vi "Tcp Request.vi"(8 "error in (no error)":errorcluster, 9 "Timeout (0ms)":i32, 11 "Conn in":refnum<k5>) -> (0 "error out":errorcluster, 2 "WSGI Request":T1, 3 "Conn out":refnum<k5>)   [LabVIEW 2021, in "HttpServer.lvlib"]
uses:
  HttpServer.lvlib
  TypeDefs/WSGI.ctl
  <vilib>/Utility/error.llb/Error Cluster From Error Code.vi
  <vilib>/ErrorRing/Error Ring.xnode
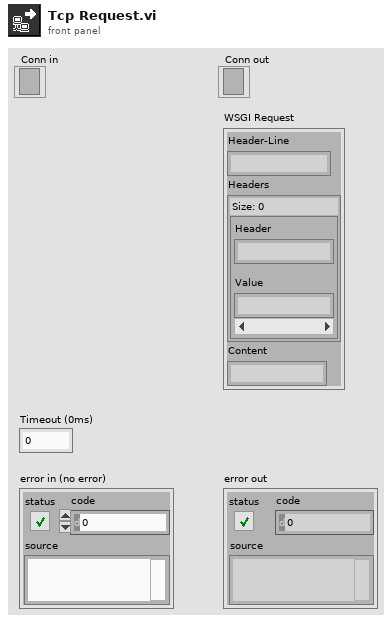
[diagram p1: front panel]
types:
  T1 = typedef "HttpServer.lvlib/WSGI.ctl" = cluster{"Header-Line":string, "Headers":map{string, string}, "Content":string}
  T2 = enum16{"Standard", "Buffered", "CRLF", "Immediate"}
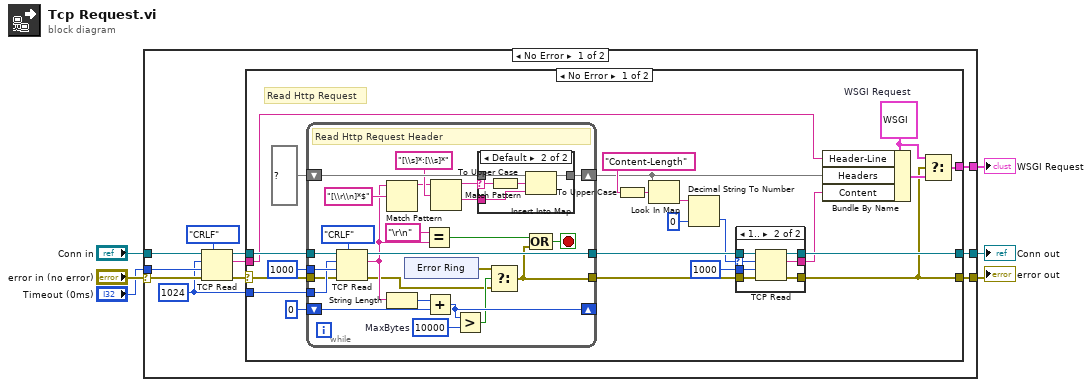
[diagram p0: block diagram]
diagram:
  n1 = case shown="No Error" "error in (no error)" {
    selector: "error in (no error)" -> [w15 w87]
    tunnel: [w17 w87] -> w6
    tunnel: [w16 w86] -> w5
    tunnel: "Conn in" -> [w12 w86]
    tunnel: "Timeout (0ms)" -> [w14 _]
    tunnel: [w13 _] -> w2
    frame No Error {
      w7 = 1024
      n2 = TCP Read(connection ID=w12, bytes to read=w7, error in (no error)=w15, 7:T2."CRLF" ("mode (standard)"), 9:w14) -> (connection ID out=w10:refnum<k5>, data out=w8:string, error out=w9:errorcluster)
      n3 = case shown="No Error" w9 {
        selector: w9 -> [w38 w85]
        tunnel: w10 -> [w39 w84]
        tunnel: w8 -> [w37 _]
        tunnel: w7 -> [w36 _]
        tunnel: [w26 w84] -> w16
        tunnel: [w19 w85] -> w17
        tunnel: [w20 _] -> w13
        frame No Error {
          w18 = T1 {"Header-Line"="", "Headers"={}, "Content"=""}  # WSGI Request
          # "Read Http Request"
          n4 = while {
            tunnel: [w55] -> w34
            tunnel: 1000 -> [w67]
            shift-right: [w65] -> w25
            shift-left: map{string, string} {} ("Map") -> [w66]
            shift-right: [w62] -> _
            shift-left: 0 -> [w63]
            tunnel: w36 -> [w54]
            tunnel: w39 -> [w73]
            tunnel: [w71] -> w35
            tunnel: w38 -> [w53]
            stop <- w68 stop-if-true
            w52 = 10000  # MaxBytes
            # "Read Http Request Header"
            n5 = TCP Read(connection ID=w73, bytes to read=w54, error in (no error)=w53, 7:T2."CRLF" ("mode (standard)"), 9:w67) -> (connection ID out=w71:refnum<k5>, data out=w57:string, error out=w49:errorcluster)
            n6 = Match Pattern(string=w57, regular expression="[\\r\\n]*$") -> (before substring=w56:string)  [unwired: 1 in, 3 out]
            n7 = String Length(string=w57) -> (length=w64:i32)
            n8 = xnode "Error Ring"() -> ("error out"=w51:errorcluster)
            n9 = Equal?(x="\r\n" ("y"), y=w57) -> (x = y?=w69:bool)
            n10 = Add(x=w64, y=w63) -> (x+y=w62:i32)
            n11 = Match Pattern(string=w56, regular expression="[\\s]*:[\\s]*") -> (before substring=w60:string, after substring=w59:string)  [unwired: 1 in, 2 out]
            n12 = Greater?(x=w62, y=w52) -> (0:w50:bool)
            n13 = case shown="Default" w60 {
              selector: w60 -> [_ w81]
              tunnel: w66 -> [w78 w83]
              tunnel: [w78 w82] -> w65
              tunnel: w59 -> [_ w80]
              frame "" {
              }
              frame Default {
                n14 = To Upper Case(1:w81) -> (0:w79:string)
                n15 = Insert Into Map(map in=w83, key=w79, value=w80) -> (map out=w82:map{string, string})  [unwired: 2 out]
              }
            }
            n16 = Select(t=w51, s=w50, f=w49) -> (s? t:f=w55:errorcluster)
            n17 = Compound Arithmetic op=OR(w69, w55) -> (w68:bool)
          }
          n18 = To Upper Case(1:"Content-Length" ("key")) -> (0:w30:string)
          n19 = Look In Map(map=w25, key=w30) -> (value=w28:string)  [unwired: 1 in, 1 out]
          n20 = Decimal String To Number(string=w28, default (0L)=0 ("default (0 I32)")) -> (number=w27:i32)  [unwired: 1 in, 1 out]
          n21 = case shown="1.." w27 {
            selector: w27 -> [_ w46]
            tunnel: w35 -> [w41 w48]
            tunnel: w34 -> [w40 w47]
            tunnel: 1000 -> [_ w45]
            tunnel: [w41 w44] -> w26
            tunnel: [w40 w43] -> w19
            tunnel: [_ w42] -> w24
            frame ..0 {
            }
            frame 1.. {
              n22 = TCP Read(connection ID=w48, bytes to read=w46, error in (no error)=w47, 9:w45) -> (connection ID out=w44:refnum<k5>, data out=w42:string, error out=w43:errorcluster)  [unwired: 1 in]
            }
          }
          n23 = Bundle By Name(cluster=w18, "Header-Line"=w37, "Headers"=w25, "Content"=w24) -> (w21:T1)
          n24 = Select(t=w18, s=w19, f=w21) -> (s? t:f=w20:T1)
        }
        frame Error {
        }
      }
    }
    frame Error {
    }
  }
  "error out" <- w6
  "Conn out" <- w5
  "WSGI Request" <- w2
